vi "Set MetaData for Stream.vi"(8 "error in":errorcluster, 9 "Ch Names":string[](array[string]), 10 "streaminfo":T1) -> (0 "error out":errorcluster)   [LabVIEW 2016, in "Lab Streaming Layer.lvlib"]
uses:
  Lab Streaming Layer.lvlib
  Custom Controls/lsl_streaminfo.ctl
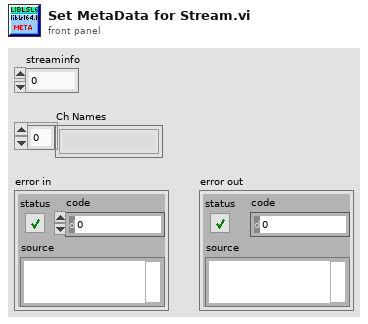
[diagram p1: front panel]
types:
  T1 = typedef "Lab Streaming Layer.lvlib/lsl_streaminfo.ctl" = u64
  T2 = typedef "Lab Streaming Layer.lvlib/lsl_xml_ptr.ctl" = u64
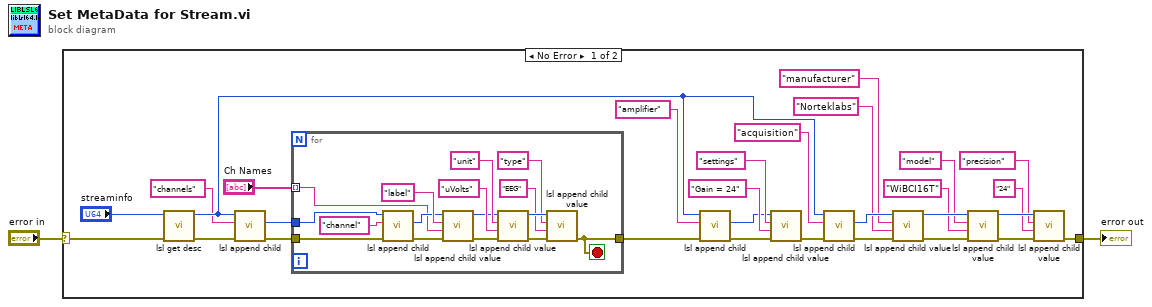
[diagram p0: block diagram]
diagram:
  n1 = case shown="No Error" "error in" {
    selector: "error in" -> [w3 w48]
    tunnel: [w31 w48] -> w2
    frame No Error {
      n2 = call "lsl get desc.vi"("error in (no error)"=w3, "streaminfo"="streaminfo") -> ("error out"=w6:errorcluster, "xml_ptr"=w22:T2)  [unwired: 8 in]
      n3 = call "lsl append child.vi"("error in (no error)"=w6, "name"="channels", "xml_ptr"=w22) -> ("error out"=w7:errorcluster, "function return"=w8:u32)  [unwired: 6 in, 1 out]
      n4 = for {
        tunnel: w7 -> [w46]
        tunnel: w8 -> [w45]
        tunnel: [w33] -> w10
        tunnel: "Ch Names" -> [w32] mode=indexing
        stop <- w33 stop-if-true
        n5 = call "lsl append child.vi"("error in (no error)"=w46, "name"="channel", "xml_ptr"=w45) -> ("error out"=w42:errorcluster, "function return"=w43:u32)  [unwired: 6 in, 1 out]
        n6 = call "lsl append child value.vi"("error in (no error)"=w42, "value"=w32, "name"="label", "xml_ptr"=w43) -> ("error out"=w35:errorcluster, "xml_ptr out"=w36:u64)  [unwired: 5 in, 1 out]
        n7 = call "lsl append child value.vi"("error in (no error)"=w35, "value"="uVolts", "name"="unit", "xml_ptr"=w36) -> ("error out"=w34:errorcluster, "xml_ptr out"=w41:u64)  [unwired: 5 in, 1 out]
        n8 = call "lsl append child value.vi"("error in (no error)"=w34, "value"="EEG", "name"="type", "xml_ptr"=w41) -> ("error out"=w33:errorcluster)  [unwired: 5 in, 2 out]
      }
      n9 = call "lsl append child.vi"("error in (no error)"=w10, "name"="amplifier", "xml_ptr"=w22) -> ("error out"=w12:errorcluster, "function return"=w13:u32)  [unwired: 6 in, 1 out]
      n10 = call "lsl append child value.vi"("error in (no error)"=w12, "value"="Gain = 24", "name"="settings", "xml_ptr"=w13) -> ("error out"=w21:errorcluster)  [unwired: 5 in, 2 out]
      n11 = call "lsl append child.vi"("error in (no error)"=w21, "name"="acquisition", "xml_ptr"=w22) -> ("error out"=w19:errorcluster, "function return"=w18:u32)  [unwired: 6 in, 1 out]
      n12 = call "lsl append child value.vi"("error in (no error)"=w19, "value"="Norteklabs", "name"="manufacturer", "xml_ptr"=w18) -> ("error out"=w29:errorcluster, "xml_ptr out"=w30:u64)  [unwired: 5 in, 1 out]
      n13 = call "lsl append child value.vi"("error in (no error)"=w29, "value"="WiBCI16T", "name"="model", "xml_ptr"=w30) -> ("error out"=w23:errorcluster, "xml_ptr out"=w28:u64)  [unwired: 5 in, 1 out]
      n14 = call "lsl append child value.vi"("error in (no error)"=w23, "value"="24", "name"="precision", "xml_ptr"=w28) -> ("error out"=w31:errorcluster)  [unwired: 5 in, 2 out]
    }
    frame Error {
    }
  }
  "error out" <- w2
